vi "DSF.Shared.Configuration.Plugin.Get Class.vi"(11 "Plugin Configuration in":refnum<class "DSF.Shared.Configuration.Plugin.lvclass">) -> (2 "class":string, 3 "Plugin Configuration out":refnum<class "DSF.Shared.Configuration.Plugin.lvclass">)   [LabVIEW 2017, in "DSF.Engine.lvlib" / "DSF.Shared.Configuration.Plugin.lvclass"]
uses:
  DSF.Shared.Configuration.Plugin.lvclass
  DSF.Shared.Configuration.Plugin.lvclass/DSF.Shared.Configuration.Plugin.ctl
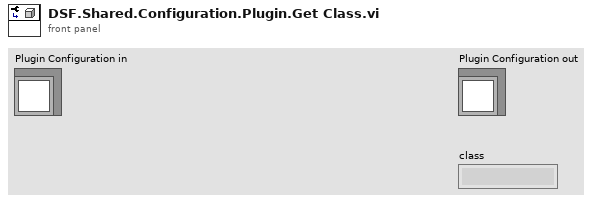
[diagram p1: front panel]
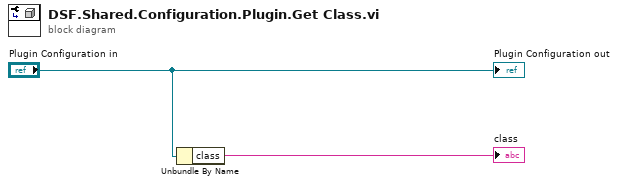
[diagram p0: block diagram]
diagram:
  n1 = Unbundle By Name("Plugin Configuration in") -> ("class"=→"class":string)
  "Plugin Configuration out" <- "Plugin Configuration in"
